vi "intialize.vi"() -> ()   [LabVIEW 2012, in "PassBouy.lvclass"]
uses:
  PassBouy.lvclass
  Data/TypeDefs/MissionTypeControl.ctl
  Data/TypeDefs/UTM Location.ctl
  PassBouy.lvclass/PassBouy.ctl
panel:
  out "PassBouy.lvclass":refnum<class "PassBouy.lvclass">
  in  "Points of Interest":T1[](array[typedef]) {"North" format="%#_10f"; "East" format="%#_8f"}
  in  "Duration (s)":dbl=-1.0
  in  "Timeout (s)":dbl=-1.0
  in  "Mission Type":T2
  out "Error Out":errorcluster
  in  "Error In":errorcluster
  in  "Tolerance (m)":dbl
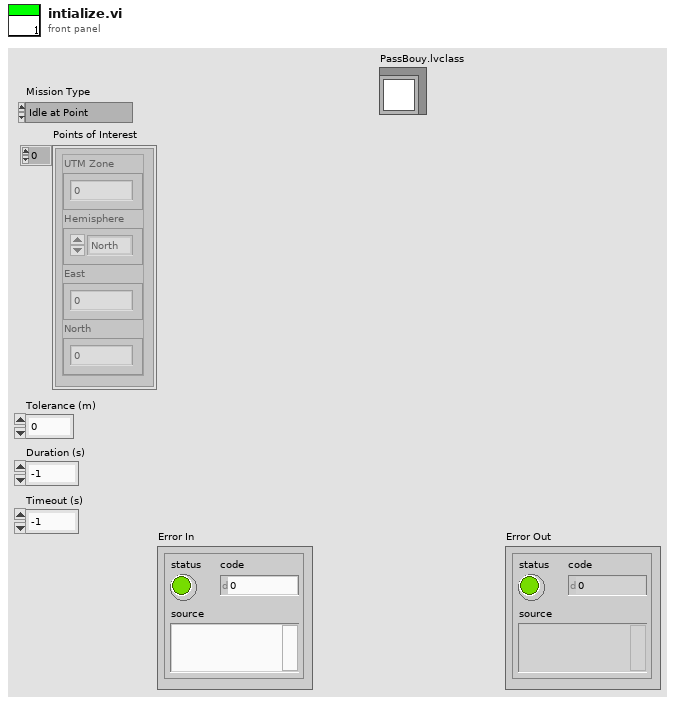
[diagram p1: front panel]
types:
  T1 = typedef "UTM Location.ctl" = cluster{"UTM Zone":dbl, "Hemisphere":enum16{"North", "South"}, "East":dbl, "North":dbl}
  T2 = typedef "MissionTypeControl.ctl" = enum16{"Idle at Point", "Drive to Waypoint", "Round Buoy to Port", "Round Buoy to Starboard", "Pass Between Buoys", "Station Keeping"}
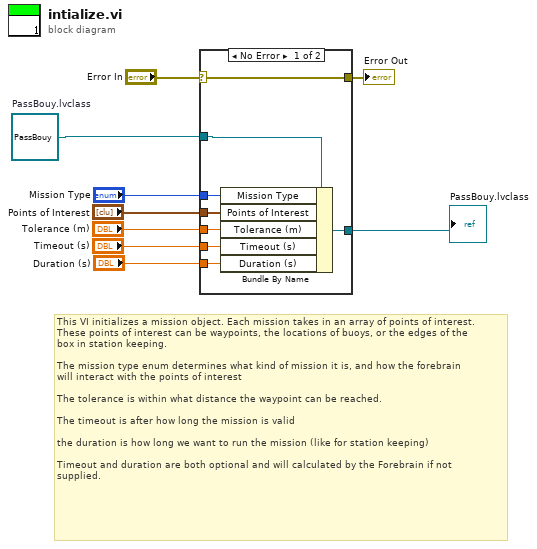
[diagram p0: block diagram]
diagram:
  w1 = refnum<class "PassBouy.lvclass"> refnum  # PassBouy.lvclass
  # "This VI initializes a mission object. Each mission takes in an array of points of interest.\nThese points of interest can be waypoints, the locations of buoys, or the edges of the \nbox in station keeping. \n\nThe mission type enum determines what kind of mission it is, and how the forebrain \nwill interact with the points of interest\n\nThe tolerance is within what distance the waypoint can be reached. \n\nThe timeout is after how long the mission is valid\n\nthe duration is how long we want to run the mission (like for station keeping)\n\nTimeout and duration are both optional and will calculated by the Forebrain if not \nsupplied."
  n1 = case shown="No Error" "Error In" {
    selector: "Error In" -> [w17 w18]
    tunnel: [w17 w18] -> w8
    tunnel: "Mission Type" -> [w16 _]
    tunnel: "Points of Interest" -> [w15 _]
    tunnel: "Tolerance (m)" -> [w14 _]
    tunnel: "Timeout (s)" -> [w13 _]
    tunnel: "Duration (s)" -> [w12 _]
    tunnel: w1 -> [w11 w19]
    tunnel: [w10 w19] -> w2
    frame No Error {
      n2 = Bundle By Name(cluster=w11, "Mission Type"=w16, "Points of Interest"=w15, "Tolerance (m)"=w14, "Timeout (s)"=w13, "Duration (s)"=w12) -> (w10:refnum<class "PassBouy.lvclass">)
    }
    frame Error {
    }
  }
  "Error Out" <- w8
  "PassBouy.lvclass" <- w2
